vi "S2C_5190CR_Proc_TcpWrite.vi"(7 "Line Seperator":string="\\n", 8 "Error In":errorcluster, 9 "Timeout(ms)":i32=5000, 10 "Data":string, 11 "Write Mode":enum16{"Normal", "Line"}(ring)) -> (0 "Error Out":errorcluster)   [LabVIEW 2015]
doc: "Performs a TCP write."
uses:
  S2C_5190CR_Proc_Globals.vi
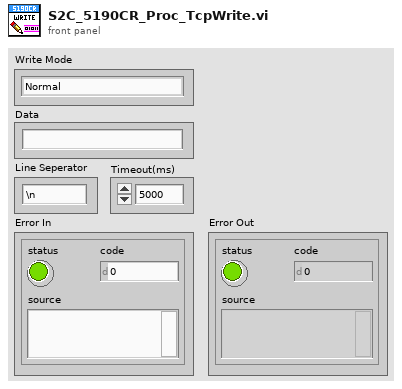
[diagram p1: front panel]
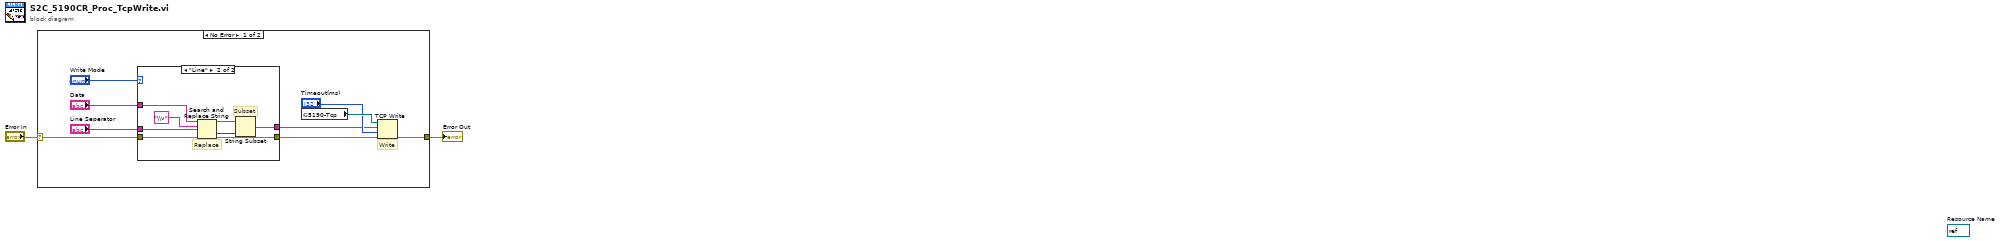
[diagram p0: block diagram]
diagram:
  (unwired) refnum<visa-resource-name> refnum  # Resource Name
  n1 = case shown="No Error" "Error In" {
    selector: "Error In" -> [w4 w22]
    tunnel: [w11 w22] -> w1
    frame No Error {
      # "Write"
      n2 = case shown="\"Line\"" "Write Mode" {
        tunnel: "Data" -> [w13 w20]
        tunnel: [w13 w14] -> w6
        tunnel: "Line Seperator" -> [_ w19]
        tunnel: w4 -> [w12 w18]
        tunnel: [w12 w17] -> w3
        frame "Normal", Default {
        }
        frame "Line" {
          # "Subset"
          # "Replace"
          n3 = Search and Replace String(input string=w20, search string="\\v", replace string=w19, error in=w18) -> (result string=w15:string, offset past replacement=w16:i32, error out=w17:errorcluster)  [unwired: 4 in, 1 out]
          n4 = String Subset(string=w15, length (rest)=w16) -> (substring=w14:string)  [unwired: 1 in]
        }
      }
      n5 = global read "S2C_5190CR_Proc_Globals.vi" "5190-Tcp"() -> (w10:refnum<k5>)
      n6 = TCP Write(connection ID=w10, data in=w6, error in (no error)=w3, 9:"Timeout(ms)") -> (error out=w11:errorcluster)  [unwired: 2 out]
    }
    frame Error {
    }
  }
  "Error Out" <- w1
